vi "SeqSet.vi"(8 "error in (no error)":errorcluster, 9 "Tag":string="No Name SEQ", 10 "Array of COR":refnum<class "Cohort.lvclass">[](array[class]), 11 "SEQ in":refnum<class "Sequence.lvclass">) -> (0 "error out":errorcluster, 3 "SEQ out":refnum<class "Sequence.lvclass">)   [LabVIEW 2012, in "Sequence.lvclass"]
uses:
  Sequence.lvclass
  Cohort.lvclass
  Sequence.lvclass/Sequence.ctl
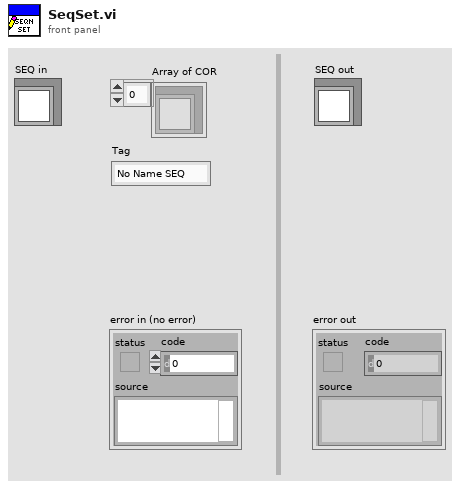
[diagram p1: front panel]
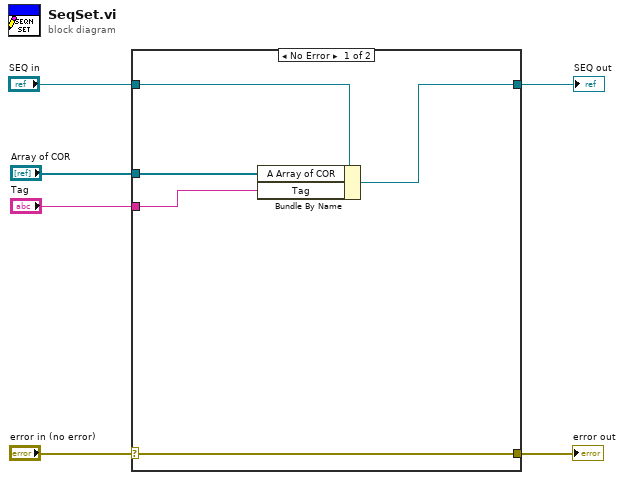
[diagram p0: block diagram]
diagram:
  n1 = case shown="No Error" "error in (no error)" {
    selector: "error in (no error)" -> [w11 w12]
    tunnel: [w11 w12] -> w5
    tunnel: [w9 w13] -> w3
    tunnel: "SEQ in" -> [w10 w13]
    tunnel: "Array of COR" -> [w8 _]
    tunnel: "Tag" -> [w7 _]
    frame No Error {
      n2 = Bundle By Name(cluster=w10, "A Array of COR"=w8, "Tag"=w7) -> (w9:refnum<class "Sequence.lvclass">)
    }
    frame Error {
    }
  }
  "error out" <- w5
  "SEQ out" <- w3
